vi "Real_assignment.vi"() -> ()   [LabVIEW 2021]
uses:
  <vilib>/addons/Fuzzy Logic/FL Fuzzy Controller (MIMO).vi
  <vilib>/addons/Fuzzy Logic/NI_Fuzzy_Logic_API.lvlib
panel:
  out "Explaination":string
  out "Turning rate":dbl
  out "Forward Velocity":dbl
  out "Left motor speed":dbl
  in  "Left motor auto switch":bool
  in  "Right motor auto switch":bool
  out "Right motor speed":dbl
  out "Object detected":bool
  out "Error":string
  in  "Right motor speed (%)":dbl(knob) scale=0.0..100.0
  out "Output sting Right":string
  in  "Path":path
  out "Right Ultrasonic (cm)":dbl(knob) scale=0.0..15.0
  out "Front Ultrasonic (cm)":dbl(knob) scale=0.0..15.0
  in  "Stop":bool
  out "Number of characters":dbl
  out "Message":string
  in  "Input string":string
  out "Proximity warning":bool
  out "Headlights":bool
  out "Light level (%)":dbl(knob) scale=0.0..100.0
  out "Left Ultrasonic (cm)":dbl(knob) scale=0.0..15.0
  out "Output sting Left":string
  in  "Left motor speed (%)":dbl(knob) scale=0.0..100.0
  # "Motor"
  # "Arduino Input"
  # "Ultrasonic sensor"
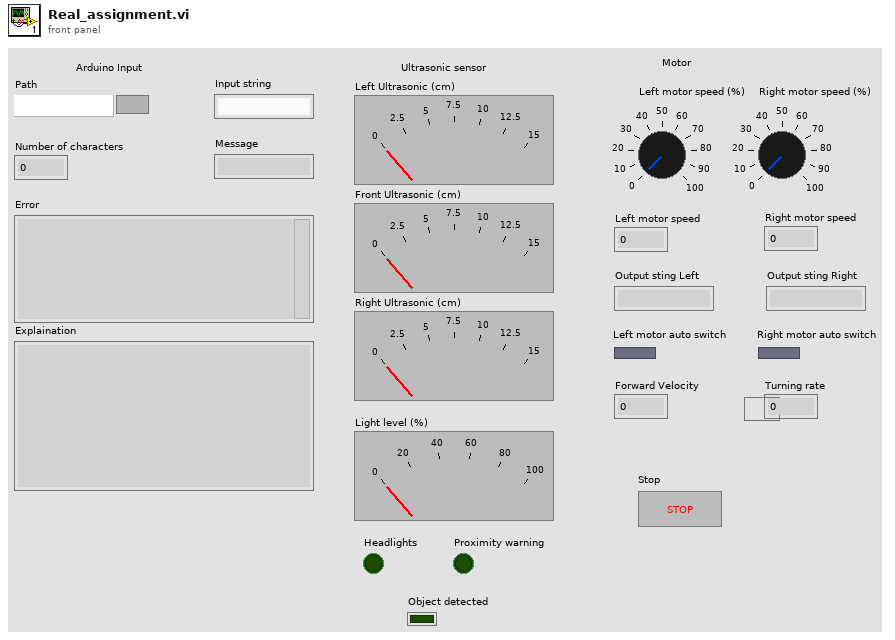
[diagram p1: front panel]
types:
  T1 = typedef "NI_Fuzzy_Logic_API.lvlib/FL System.ctl" = cluster{"input variables":T2[], "output variables":T2[], "rules":T5[], "defuzzification method":T11, "description":string, "user MF interpolating polynomials":T12[]}
  T2 = typedef "NI_Fuzzy_Logic_API.lvlib/FL Variable.ctl" = cluster{"name":string, "range":dbl[], "MFs":T3[]}
  T3 = typedef "NI_Fuzzy_Logic_API.lvlib/FL Membership Function.ctl" = cluster{"name":string, "shape":T4, "points":dbl[], "color":u32, "user-defined shape index":i32}
  T4 = typedef "NI_Fuzzy_Logic_API.lvlib/FL Membership Function Shape.ctl" = u16
  T5 = typedef "NI_Fuzzy_Logic_API.lvlib/FL Rule.ctl" = cluster{"antecedents":T6[], "antecedent connective":T8, "consequents":T9[], "consequent implication":T10, "degree of support":dbl}
  T6 = typedef "NI_Fuzzy_Logic_API.lvlib/FL Antecedent.ctl" = cluster{"Var Index":i32, "MF Index":i32, "Cond":T7}
  T7 = typedef "NI_Fuzzy_Logic_API.lvlib/FL Modifier.ctl" = u16
  T8 = typedef "NI_Fuzzy_Logic_API.lvlib/FL Antecedent Connective.ctl" = u16
  T9 = typedef "NI_Fuzzy_Logic_API.lvlib/FL Consequent.ctl" = cluster{"Var Index":i32, "MF Index":i32, "Cond":T7}
  T10 = typedef "NI_Fuzzy_Logic_API.lvlib/FL Consequent Implication.ctl" = u16
  T11 = typedef "NI_Fuzzy_Logic_API.lvlib/FL Defuzzification.ctl" = u16
  T12 = typedef "NI_Fuzzy_Logic_API.lvlib/FL Interpolating polynomials.ctl" = cluster{"X":dbl[], "Y":dbl[], "Y(x) coeff":dbl[][], "X(y) coeff":dbl[][], "Area(y) coeff":dbl[][], "coa_x(y) coeff":dbl[][]}
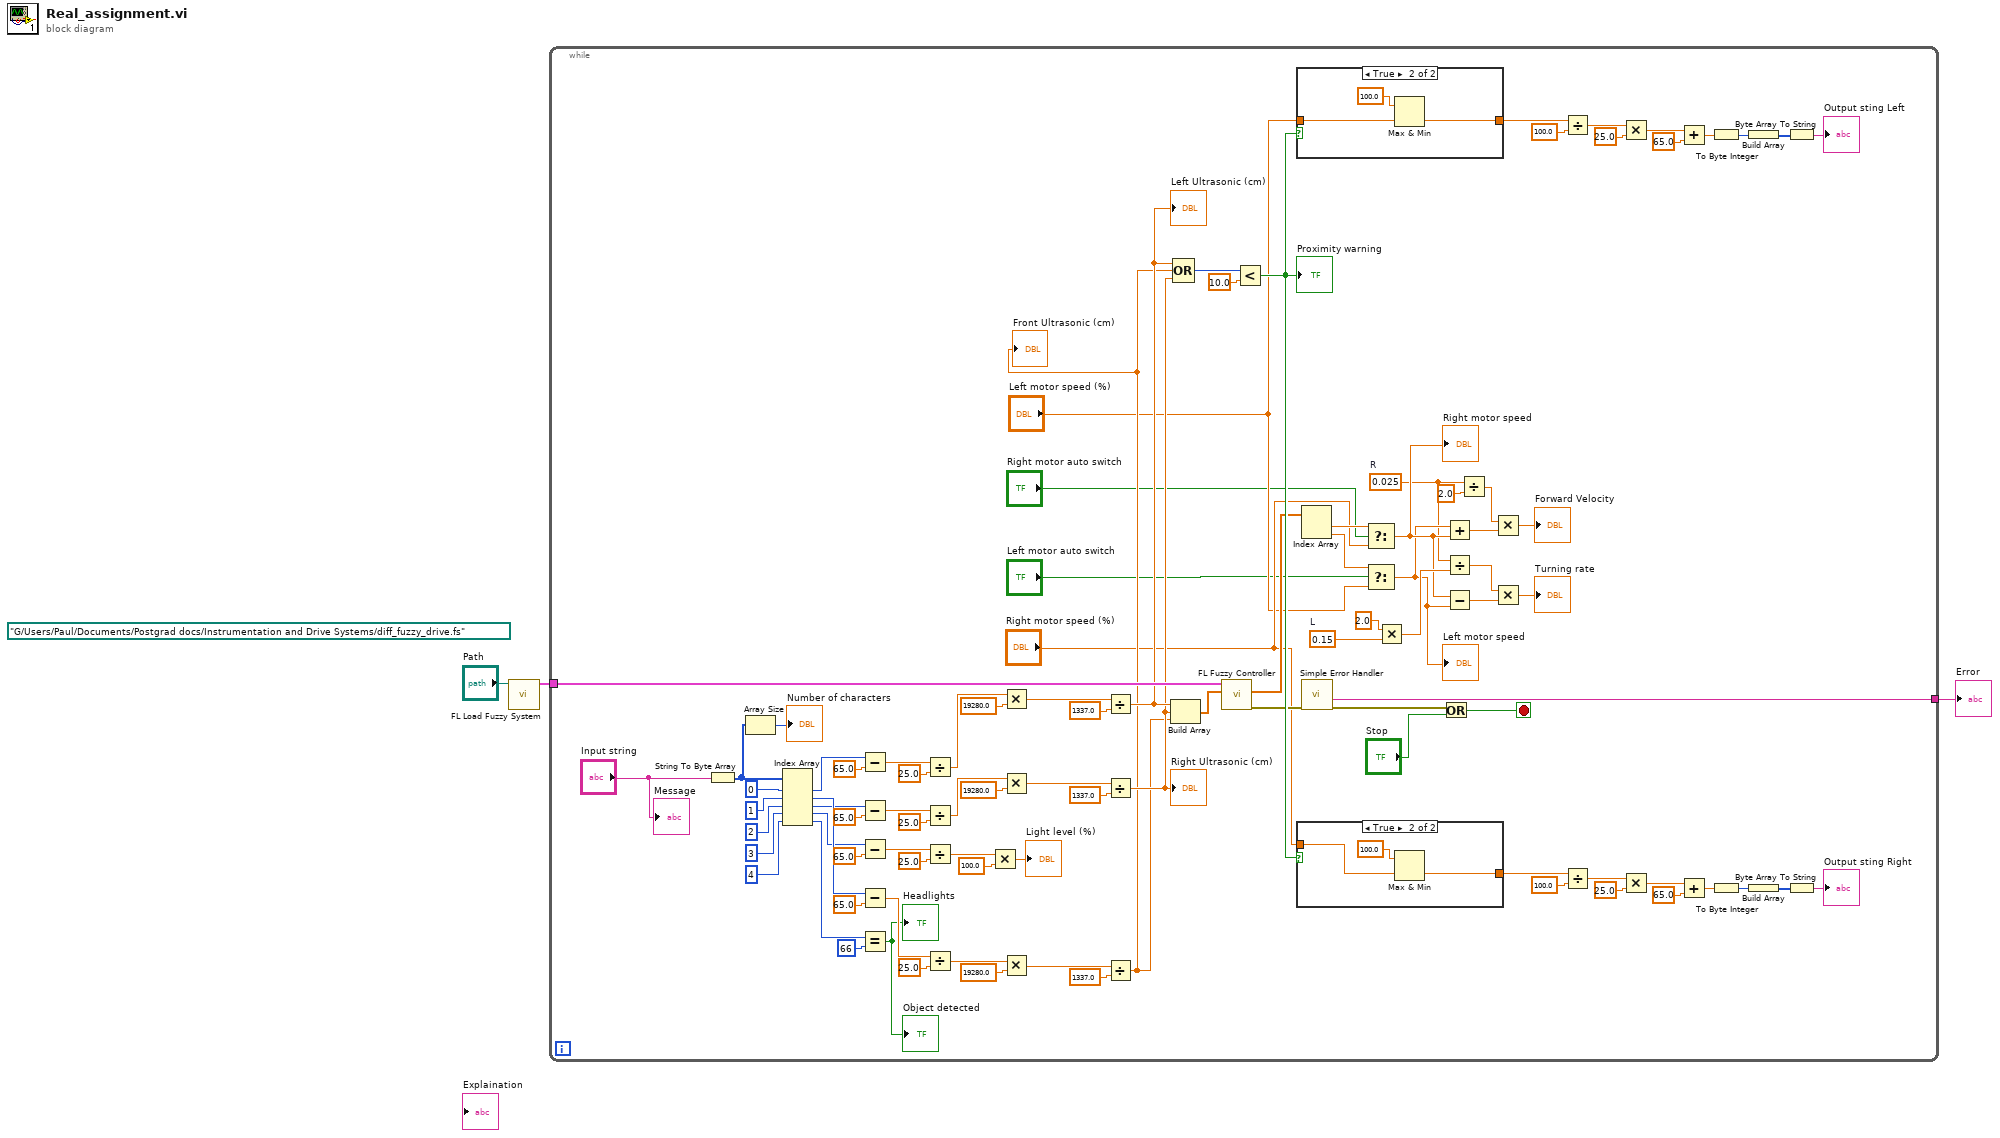
[diagram p0: block diagram]
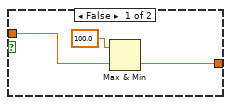
[diagram p2: hidden frame]
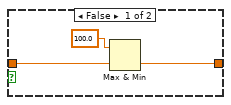
[diagram p3: hidden frame]
diagram:
  (unwired) path "G:/Users/Paul/Documents/Postgrad docs/Instrumentation and Drive Systems/diff_fuzzy_drive.fs" ("Path")
  n1 = call <vilib>:"FL Load Fuzzy System.vi"("file path"="Path") -> ("fuzzy system out"=w2:T1)  [unwired: 9 in, 1 out]
  n2 = while {
    tunnel: w2 -> [w32]
    tunnel: [w30] -> w1
    stop <- w34 stop-if-true
    w5 = 0.15  # L
    w7 = 0.025  # R
    n3 = String To Byte Array(string="Input string") -> (unsigned byte array=w96:u8[])
    n4 = Array Size(array=w96) -> (size(s)=→"Number of characters":i32)
    n5 = Index Array(array=w96, index #1=0, index #2=1, index #3=2, index #4=3, index #5=4) -> (element #1=w92:u8, element #2=w51:u8, element #3=w50:u8, element #4=w49:u8, element #5=w48:u8)
    n6 = Subtract(x=w92, y=65.0) -> (x-y=w90:dbl)
    n7 = Subtract(x=w50, y=65.0) -> (x-y=w57:dbl)
    n8 = Subtract(x=w49, y=65.0) -> (x-y=w83:dbl)
    n9 = Subtract(x=w51, y=65.0) -> (x-y=w64:dbl)
    n10 = Equal?(x=w48, y=66) -> (x = y?=→"Headlights" →"Object detected":bool)
    n11 = Divide(x=w90, y=25.0) -> (x/y=w88:dbl)
    n12 = Divide(x=w57, y=25.0) -> (x/y=w55:dbl)
    n13 = Divide(x=w83, y=25.0) -> (x/y=w81:dbl)
    n14 = Divide(x=w64, y=25.0) -> (x/y=w62:dbl)
    n15 = Multiply(x=w81, y=100.0) -> (x*y=→"Light level (%)":dbl)
    n16 = Multiply(x=w88, y=19280.0) -> (x*y=w86:dbl)
    n17 = Multiply(x=w55, y=19280.0) -> (x*y=w53:dbl)
    n18 = Multiply(x=w62, y=19280.0) -> (x*y=w60:dbl)
    n19 = Divide(x=w86, y=1337.0) -> (x/y=w26:dbl)
    "Left Ultrasonic (cm)" <- w26
    n20 = Divide(x=w53, y=1337.0) -> (x/y=w25:dbl)
    "Right Ultrasonic (cm)" <- w25
    n21 = Divide(x=w60, y=1337.0) -> (x/y=w24:dbl)
    "Front Ultrasonic (cm)" <- w24
    n22 = Build Array(w26, w25, w24) -> (w23:dbl[])
    n23 = Compound Arithmetic op=OR(w26, w24, w25) -> (w47:i32)
    n24 = call-poly <vilib>:"FL Fuzzy Controller.vi"("input values"=w23, "fuzzy system in"=w32) -> ("error out"=w31:errorcluster, "output values"=w27:dbl[])  [unwired: 5 in, 3 out]
    n25 = Less?(x=w47, y=10.0) -> (x < y?=w36:bool)
    "Proximity warning" <- w36
    n26 = case shown="True" w36 {
      tunnel: "Left motor speed (%)" -> [w105 w109]
      tunnel: [w106 w108] -> w76
      frame False {
        n27 = Max & Min(x=100.0, y=w105) -> (min(x,y)=w106:dbl)  [unwired: 1 out]
      }
      frame True {
        n28 = Max & Min(x=100.0, y=w109) -> (min(x,y)=w108:dbl)  [unwired: 1 out]
      }
    }
    n29 = case shown="True" w36 {
      tunnel: [w100 w103] -> w37
      tunnel: "Right motor speed (%)" -> [w99 w102]
      frame False {
        n30 = Max & Min(x=100.0, y=w99) -> (min(x,y)=w100:dbl)  [unwired: 1 out]
      }
      frame True {
        n31 = Max & Min(x=100.0, y=w102) -> (min(x,y)=w103:dbl)  [unwired: 1 out]
      }
    }
    n32 = Index Array(array=w27) -> (element #1=w22:dbl, element #2=w20:dbl)  [unwired: 2 in]
    n33 = call <vilib>:"Simple Error Handler.vi"("error in (no error)"=w31) -> ("source out"=w30:string, "error out"=w29:errorcluster)  [unwired: 4 in, 3 out]
    n34 = Select(t=w22, s="Right motor auto switch", f="Right motor speed (%)") -> (s? t:f=w11:dbl)
    "Right motor speed" <- w11
    n35 = Select(t=w20, s="Left motor auto switch", f="Left motor speed (%)") -> (s? t:f=w8:dbl)
    "Left motor speed" <- w8
    n36 = Multiply(x=2.0, y=w5) -> (x*y=w12:dbl)
    n37 = Or(x=w29, y="Stop") -> (x .or. y?=w34:bool)
    n38 = Add(x=w8, y=w11) -> (x+y=w14:dbl)
    n39 = Divide(x=w7, y=w12) -> (x/y=w10:dbl)
    n40 = Subtract(x=w11, y=w8) -> (x-y=w9:dbl)
    n41 = Divide(x=w7, y=2.0) -> (x/y=w15:dbl)
    n42 = Multiply(x=w15, y=w14) -> (x*y=→"Forward Velocity":dbl)
    n43 = Multiply(x=w10, y=w9) -> (x*y=→"Turning rate":dbl)
    n44 = Divide(x=w76, y=100.0) -> (x/y=w75:dbl)
    n45 = Divide(x=w37, y=100.0) -> (x/y=w45:dbl)
    n46 = Multiply(x=w75, y=25.0) -> (x*y=w77:dbl)
    n47 = Multiply(x=w45, y=25.0) -> (x*y=w46:dbl)
    n48 = Add(x=w77, y=65.0) -> (x+y=w71:dbl)
    n49 = Add(x=w46, y=65.0) -> (x+y=w41:dbl)
    n50 = To Byte Integer(number=w71) -> (8bit integer=w70:i8)
    n51 = To Byte Integer(number=w41) -> (8bit integer=w40:i8)
    n52 = Build Array(w70) -> (w69:i8[])
    n53 = Build Array(w40) -> (w39:i8[])
    n54 = Byte Array To String(unsigned byte array=w69) -> (string=→"Output sting Left":string)
    n55 = Byte Array To String(unsigned byte array=w39) -> (string=→"Output sting Right":string)
    "Message" <- "Input string"
  }
  "Error" <- w1
